vi "PUB-SUB.vi"() -> ()   [LabVIEW 2018]
uses:
  RxTx/CM_RxTx.lvclass
  socket PUB/socket PUB.lvclass
  C:/Users/Denis/Desktop/communication-manager/communication-manager/Socket/Socket.lvclass
  socket SUB/socket SUB.lvclass
  Socket/Socket.lvclass
  <vilib>/addons/zeromq/zmq_context.lvclass
panel:
  in  "log file path":path=path "C:/Users/Denis/Desktop/communication-manager/communication-manager/CFG file"
  out "error out 3":errorcluster
  in  "Queue RX 2":refnum<class "CM_RxTx.lvclass">
  out "Received message":string
  in  "socket SUB.lvclass":refnum<class "socket SUB.lvclass">
  in  "socket PUB.lvclass":refnum<class "socket PUB.lvclass">
  in  "message":string
  in  "send":bool
  out "error out 2":errorcluster
  in  "Queue RX":refnum<class "CM_RxTx.lvclass">
  in  "stop":bool
  # "PUB endpoint"
  # "SUB endpoint"
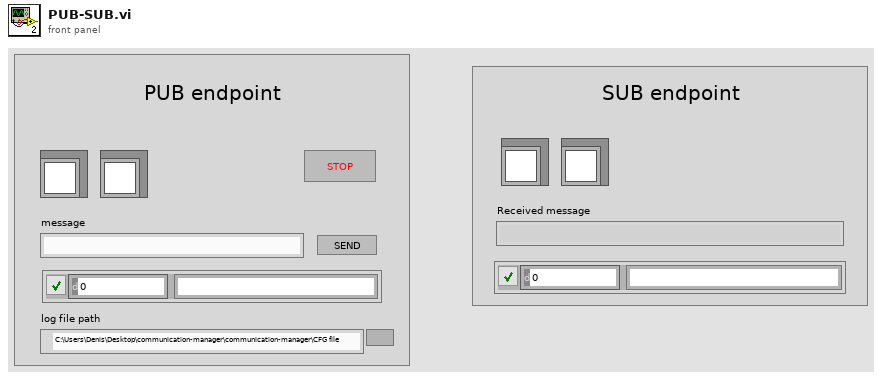
[diagram p1: front panel]
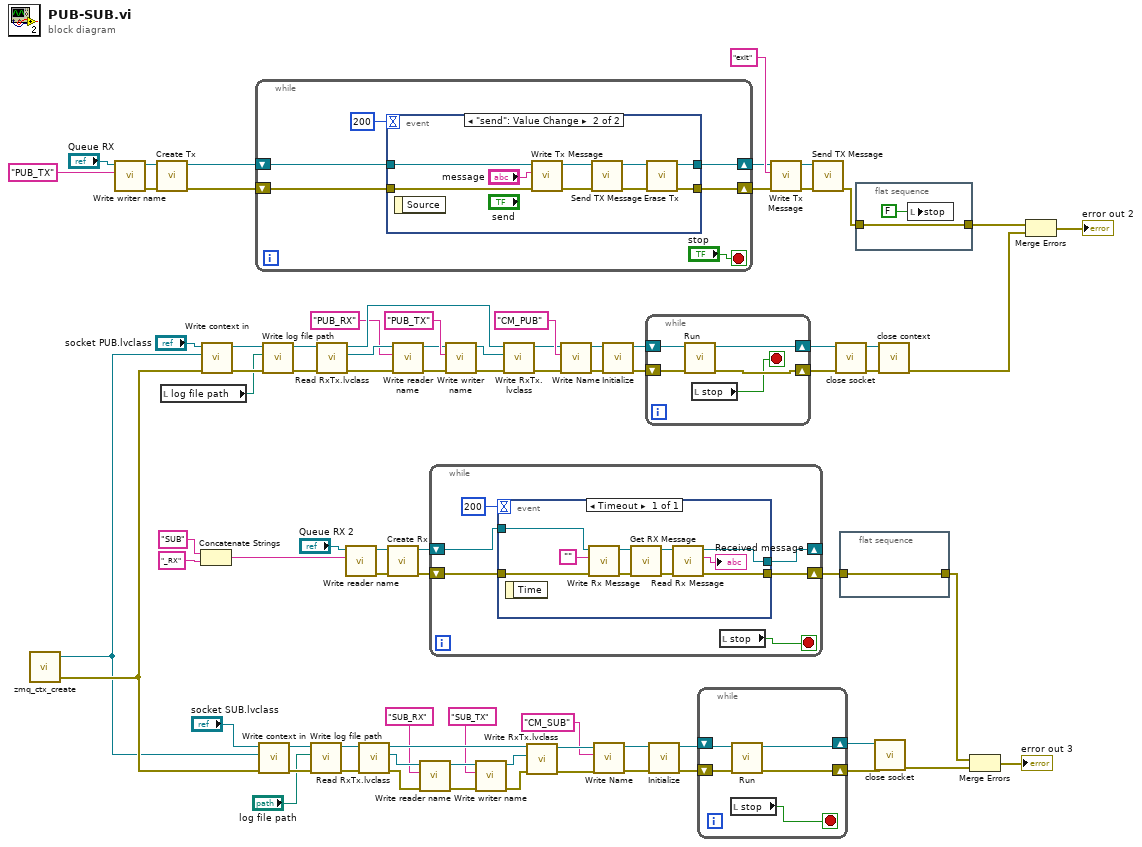
[diagram p0: block diagram]
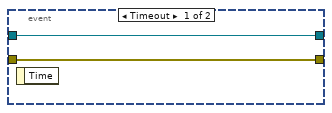
[diagram p2: hidden frame]
diagram:
  n1 = call <vilib>:"zmq_ctx_create.vi"() -> ("error out"=w28:errorcluster, "context out"=w27:refnum<class "zmq_context.lvclass">)  [unwired: 4 in]
  n2 = call-dynamic "Write writer name.vi"("Tx name"="PUB_TX", "RxTx in"="Queue RX") -> ("error out"=w76:errorcluster, "RxTx out"=w77:refnum<class "CM_RxTx.lvclass">)  [unwired: 8 in]
  n3 = call "Create Tx.vi"("error in (no error)"=w76, "RxTx in"=w77) -> ("error out"=w75:errorcluster, "RxTx out"=w79:refnum<class "CM_RxTx.lvclass">)  [unwired: 8 in]
  n4 = local read "log file path"() -> (w1:path)
  n5 = Concatenate Strings("SUB" ("string"), "_RX" ("string")) -> (w17:string)
  n6 = call-dynamic "Write context in.vi"("error in (no error)"=w28, "zeromq.lvlib:ZeroMQ Context"=w27, "Socket in"="socket PUB.lvclass") -> ("error out"=w7:errorcluster, "Socket out"=w10:refnum<class "socket PUB.lvclass">)  [unwired: 7 in]
  n7 = while {
    shift-right: [w82] -> w50
    shift-left: w79 -> [w84]
    shift-right: [w81] -> w47
    shift-left: w75 -> [w83]
    stop <- "stop" stop-if-true
    n8 = event shown="[1] \"send\": Value Change" {
      selector: _ -> [_ _]
      dyn-events: _ -> [_ _]
      timeout: 200 -> [_ _]
      tunnel: [w87 w93] -> w82
      tunnel: [w86 w92] -> w81
      tunnel: w84 -> [w87 w89]
      tunnel: w83 -> [w86 w88]
      event Timeout {
        n9 = event-data() -> ()  [unwired: 1 in, 1 out]
      }
      event "send": Value Change {
        n10 = event-data() -> ()  [unwired: 1 in, 1 out]
        n11 = call "Write Tx Message.vi"("error in (no error)"=w88, "Tx Message"="message", "RxTx in"=w89) -> ("error out"=w90:errorcluster, "RxTx out"=w95:refnum<class "CM_RxTx.lvclass">)  [unwired: 7 in]
        n12 = call "Send TX Message.vi"("error in (no error)"=w90, "RxTx in"=w95) -> ("error out"=w91:errorcluster, "RxTx out"=w94:refnum<class "CM_RxTx.lvclass">)  [unwired: 8 in]
        n13 = call "Erase Tx.vi"("error in (no error)"=w91, "RxTx in"=w94) -> ("error out"=w92:errorcluster, "RxTx out"=w93:refnum<class "CM_RxTx.lvclass">)  [unwired: 8 in]
      }
    }
  }
  n14 = call-dynamic "Write context in.vi"("error in (no error)"=w28, "zeromq.lvlib:ZeroMQ Context"=w27, "Socket in"="socket SUB.lvclass") -> ("error out"=w6:errorcluster, "Socket out"=w3:refnum<class "socket SUB.lvclass">)  [unwired: 7 in]
  n15 = call-dynamic "Write log file path.vi"("error in (no error)"=w7, "log file path"=w1, "Socket in"=w10) -> ("error out"=w8:errorcluster, "Socket out"=w9:refnum<class "socket PUB.lvclass">)  [unwired: 7 in]
  n16 = call-dynamic "Write log file path.vi"("error in (no error)"=w6, "log file path"="log file path", "Socket in"=w3) -> ("error out"=w4:errorcluster, "Socket out"=w5:refnum<class "socket SUB.lvclass">)  [unwired: 7 in]
  n17 = call-dynamic "Read RxTx.lvclass.vi"("error in (no error)"=w8, "Socket in"=w9) -> ("error out"=w66:errorcluster, "RxTx.lvclass"=w70:refnum<class "CM_RxTx.lvclass">, "Socket out"=w67:refnum<class "socket PUB.lvclass">)  [unwired: 7 in]
  n18 = call-dynamic "Write reader name.vi"("RX name"=w17, "RxTx in"="Queue RX 2") -> ("error out"=w19:errorcluster, "RxTx out"=w20:refnum<class "CM_RxTx.lvclass">)  [unwired: 8 in]
  n19 = call-dynamic "Read RxTx.lvclass.vi"("error in (no error)"=w4, "Socket in"=w5) -> ("error out"=w38:errorcluster, "RxTx.lvclass"=w34:refnum<class "CM_RxTx.lvclass">, "Socket out"=w37:refnum<class "socket SUB.lvclass">)  [unwired: 7 in]
  n20 = call "Create Rx.vi"("error in (no error)"=w19, "RxTx in"=w20) -> ("error out"=w18:errorcluster, "RxTx out"=w21:refnum<class "CM_RxTx.lvclass">)  [unwired: 8 in]
  n21 = call-dynamic "Write reader name.vi"("error in (no error)"=w66, "RX name"="PUB_RX" ("reader name"), "RxTx in"=w70) -> ("error out"=w65:errorcluster, "RxTx out"=w69:refnum<class "CM_RxTx.lvclass">)  [unwired: 7 in]
  n22 = call-dynamic "Write reader name.vi"("error in (no error)"=w38, "RX name"="SUB_RX" ("reader name"), "RxTx in"=w34) -> ("error out"=w39:errorcluster, "RxTx out"=w35:refnum<class "CM_RxTx.lvclass">)  [unwired: 7 in]
  n23 = while {
    shift-right: [w100] -> _
    shift-left: w21 -> [w101]
    shift-right: [w98] -> w14
    shift-left: w18 -> [w99]
    stop <- w97 stop-if-true
    n24 = event shown="[0] Timeout" {
      selector: _ -> [_]
      dyn-events: _ -> [_]
      timeout: 200 -> [_]
      tunnel: w101 -> [w109]
      tunnel: [w107] -> w100
      tunnel: w99 -> [w104]
      tunnel: [w103] -> w98
      event Timeout {
        n25 = event-data() -> ()  [unwired: 1 in, 1 out]
        n26 = call "Write Rx Message.vi"("error in (no error)"=w104, "Rx Message"="", "RxTx in"=w109) -> ("error out"=w106:errorcluster, "RxTx out"=w108:refnum<class "CM_RxTx.lvclass">)  [unwired: 7 in]
        n27 = call "Get RX Message.vi"("error in (no error)"=w106, "RxTx in"=w108) -> ("error out"=w110:errorcluster, "RxTx out"=w112:refnum<class "CM_RxTx.lvclass">)  [unwired: 7 in, 1 out]
        n28 = call "Read Rx Message.vi"("error in (no error)"=w110, "RxTx in"=w112) -> ("error out"=w103:errorcluster, "Rx Message"=→"Received message":string, "RxTx out"=w107:refnum<class "CM_RxTx.lvclass">)  [unwired: 7 in]
      }
    }
    n29 = local read "stop"() -> (w97:bool)
  }
  n30 = call-dynamic "Write writer name.vi"("error in (no error)"=w65, "Tx name"="PUB_TX" ("writer name"), "RxTx in"=w69) -> ("error out"=w64:errorcluster, "RxTx out"=w68:refnum<class "CM_RxTx.lvclass">)  [unwired: 7 in]
  n31 = call-dynamic "Write writer name.vi"("error in (no error)"=w39, "Tx name"="SUB_TX" ("writer name"), "RxTx in"=w35) -> ("error out"=w40:errorcluster, "RxTx out"=w36:refnum<class "CM_RxTx.lvclass">)  [unwired: 7 in]
  n32 = call-dynamic "Write RxTx.lvclass.vi"("error in (no error)"=w64, "RxTx.lvclass"=w68, "Socket in"=w67) -> ("error out"=w54:errorcluster, "Socket out"=w55:refnum<class "socket PUB.lvclass">)  [unwired: 7 in]
  n33 = call-dynamic "Write RxTx.lvclass.vi"("error in (no error)"=w40, "RxTx.lvclass"=w36, "Socket in"=w37) -> ("error out"=w43:errorcluster, "Socket out"=w42:refnum<class "socket SUB.lvclass">)  [unwired: 7 in]
  n34 = call-dynamic "Write Name.vi"("error in (no error)"=w54, "Name"="CM_PUB", "Socket in"=w55) -> ("error out"=w62:errorcluster, "Socket out"=w63:refnum<class "socket PUB.lvclass">)  [unwired: 7 in]
  n35 = call-dynamic "Write Name.vi"("error in (no error)"=w43, "Name"="CM_SUB", "Socket in"=w42) -> ("error out"=w29:errorcluster, "Socket out"=w30:refnum<class "socket SUB.lvclass">)  [unwired: 7 in]
  n36 = call-dynamic "Initialize.vi"("error in (no error)"=w62, "socket PUB in"=w63) -> ("error out"=w59:errorcluster, "socket PUB out"=w61:refnum<class "socket PUB.lvclass">)  [unwired: 8 in]
  n37 = while {
    shift-right: [w115] -> w60
    shift-left: w61 -> [w117]
    shift-right: [w114] -> w58
    shift-left: w59 -> [w116]
    stop <- w113 stop-if-true
    n38 = call-dynamic "Run.vi"("error in (no error)"=w116, "socket PUB in"=w117) -> ("error out"=w114:errorcluster, "socket PUB out"=w115:refnum<class "socket PUB.lvclass">)  [unwired: 8 in]
    n39 = local read "stop"() -> (w113:bool)
  }
  n40 = call-dynamic "Initialize.vi"("error in (no error)"=w29, "socket SUB in"=w30) -> ("error out"=w25:errorcluster, "socket SUB out"=w26:refnum<class "socket SUB.lvclass">)  [unwired: 8 in]
  n41 = while {
    shift-right: [w120] -> w23
    shift-left: w26 -> [w122]
    shift-right: [w119] -> w24
    shift-left: w25 -> [w121]
    stop <- w118 stop-if-true
    n42 = local read "stop"() -> (w118:bool)
    n43 = call-dynamic "Run.vi"("error in (no error)"=w121, "socket SUB in"=w122) -> ("error out"=w119:errorcluster, "socket SUB out"=w120:refnum<class "socket SUB.lvclass">)  [unwired: 8 in]
  }
  n44 = call "Write Tx Message.vi"("error in (no error)"=w47, "Tx Message"="exit" ("Publication 2"), "RxTx in"=w50) -> ("error out"=w48:errorcluster, "RxTx out"=w51:refnum<class "CM_RxTx.lvclass">)  [unwired: 7 in]
  n45 = call "Send TX Message.vi"("error in (no error)"=w48, "RxTx in"=w51) -> ("error out"=w49:errorcluster)  [unwired: 8 in, 1 out]
  n46 = call "close socket.vi"("error in (no error)"=w58, "Socket in"=w60) -> ("error out"=w73:errorcluster, "Socket out"=w72:refnum<class "socket PUB.lvclass">)  [unwired: 8 in]
  n47 = flat-sequence {
    tunnel: w14 -> [w123]
    tunnel: [w123] -> w13
    frame #0 {
    }
  }
  n48 = flat-sequence {
    tunnel: w49 -> [w125]
    tunnel: [w125] -> w46
    frame #0 {
      n49 = local write "stop"(FALSE ("stop")) -> ()
    }
  }
  n50 = call "close socket.vi"("error in (no error)"=w24, "Socket in"=w23) -> ("error out"=w12:errorcluster)  [unwired: 8 in, 1 out]
  n51 = call-dynamic "close context.vi"("error in (no error)"=w73, "Socket in"=w72) -> ("error out"=w44:errorcluster)  [unwired: 8 in, 1 out]
  n52 = Merge Errors(w13, w12) -> (→"error out 3":errorcluster)
  n53 = Merge Errors(w46, w44) -> (→"error out 2":errorcluster)
